vi "getScanKey.vi"(8 "error in (no error)":errorcluster, 11 "Experiment in":refnum<class "Experiment.lvclass">) -> (0 "error out":errorcluster, 2 "Scan Key":T1, 3 "Experiment out":refnum<class "Experiment.lvclass">)   [LabVIEW 2016, in "Experiment.lvclass"]
uses:
  Experiment.lvclass
  Experiment.lvclass/Experiment.ctl
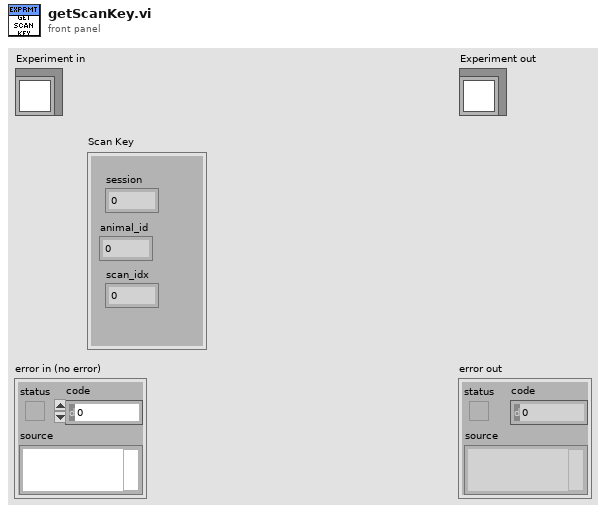
[diagram p1: front panel]
types:
  T1 = cluster{"session":dbl, "animal_id":dbl, "scan_idx":dbl}
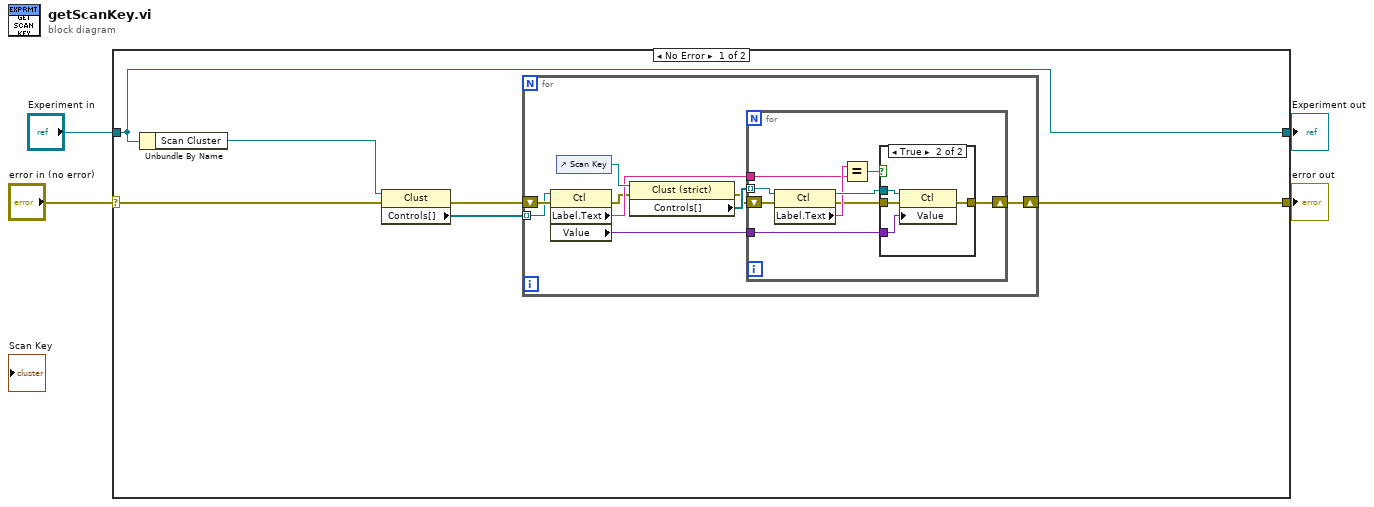
[diagram p0: block diagram]
diagram:
  n1 = case shown="No Error" "error in (no error)" {
    selector: "error in (no error)" -> [w6 w35]
    tunnel: [w9 w35] -> w3
    tunnel: "Experiment in" -> [w10 w34]
    tunnel: [w10 w34] -> w1
    frame No Error {
      n2 = Unbundle By Name(w10) -> ("Scan Cluster"=w5:refnum<vi>)
      n3 = property class="Clust"(reference=w5, error in=w6) -> (error out=w8:errorcluster, "Controls[]"=w7:refnum<vi>[])  [unwired: 1 out]
      n4 = for {
        shift-right: [w14] -> w9
        shift-left: w8 -> [w19]
        tunnel: w7 -> [w11] mode=indexing
        n5 = property class="Ctl"(reference=w11, error in=w19) -> (error out=w13:errorcluster, "Label.Text"=w16:string, "Value"=w15:variant)  [unwired: 1 out]
        n6 = control-ref of="Scan Key"() -> (w17:refnum<vi>)
        n7 = property class="Clust (strict)"(reference=w17, error in=w13) -> (error out=w12:errorcluster, "Controls[]"=w18:refnum<vi>[])  [unwired: 1 out]
        n8 = for {
          tunnel: w18 -> [w28] mode=indexing
          shift-right: [w22] -> w14
          shift-left: w12 -> [w24]
          tunnel: w16 -> [w21]
          tunnel: w15 -> [w20]
          n9 = property class="Ctl"(reference=w28, error in=w24) -> (reference out=w27:refnum<vi>, error out=w23:errorcluster, "Label.Text"=w25:string)
          n10 = Equal?(x=w25, y=w21) -> (x = y?=w26:bool)
          n11 = case shown="True" w26 {
            tunnel: w27 -> [_ w33]
            tunnel: w23 -> [w29 w32]
            tunnel: [w29 w31] -> w22
            tunnel: w20 -> [_ w30]
            frame False {
            }
            frame True {
              n12 = property class="Ctl"(reference=w33, error in=w32, "Value"=w30) -> (error out=w31:errorcluster)  [unwired: 1 out]
            }
          }
        }
      }
    }
    frame Error {
    }
  }
  "error out" <- w3
  "Experiment out" <- w1
